vi "Configure Data Output Format.vi"(8 "error in (no error)":errorcluster, 9 "Byte Order (1: Little Endian)":i32(ring)=1 items=["Big Endian", "Little Endian"], 10 "Data Precision (6)":i32=6, 11 "VISA resource name":refnum<visa-resource-name>) -> (0 "error out":errorcluster, 3 "VISA resource name out":refnum<visa-resource-name>)   [LabVIEW 2020, in "Keithley 2600 Series.lvlib"]
doc: "Configures the format of the output data."
uses:
  <instrlib>/Keithley 2600 Series/Keithley 2600 Series.lvlib
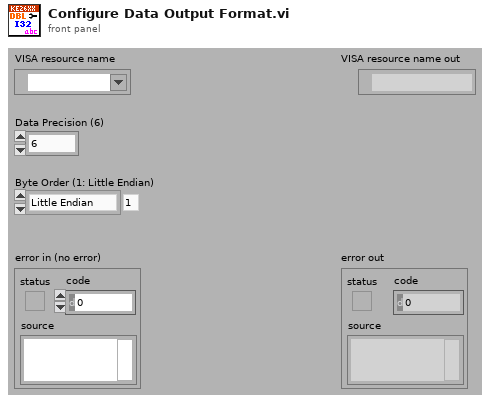
[diagram p1: front panel]
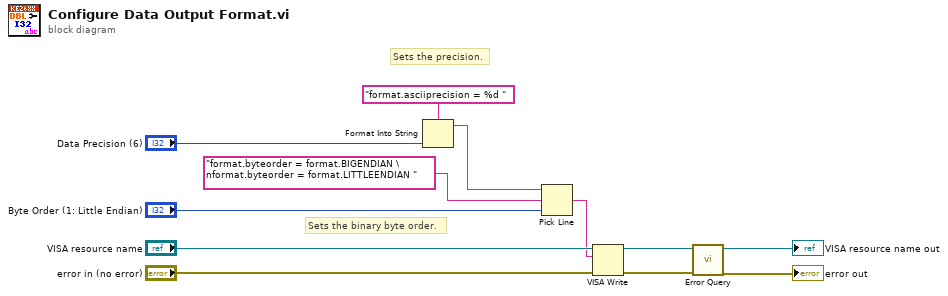
[diagram p0: block diagram]
diagram:
  # "Sets the precision."
  # "Sets the binary byte order."
  n1 = Format Into String(format string="format.asciiprecision = %d ", "Data Precision (6)") -> (resulting string=w2:string)  [unwired: 2 in, 1 out]
  n2 = Pick Line(string ("")=w2, multi-line string="format.byteorder = format.BIGENDIAN \nformat.byteorder = format.LITTLEENDIAN ", line index="Byte Order (1: Little Endian)") -> (output string=w1:string)
  n3 = VISA Write(VISA resource name="VISA resource name", write buffer=w1, error in (no error)="error in (no error)") -> (VISA resource name out=w6:refnum<visa-resource-name>, error out=w5:errorcluster)  [unwired: 1 out]
  n4 = call <instrlib>:"Error Query.vi"("error in (no error)"=w5, "VISA resource name"=w6) -> ("error out"=→"error out":errorcluster, "VISA resource name out"=→"VISA resource name out":refnum<visa-resource-name>)  [unwired: 6 in, 2 out]
